vi "CloseNode.vi"(8 "error in":errorcluster, 11 "node ref":T1) -> (0 "error out":errorcluster)   [LabVIEW 2013, in "NISE_CEF_TreeControl.lvlib"]
doc: "This is the node Clean Up Vi it will close all the open references for the node and its childs"
uses:
  NISE_CEF_TreeControl.lvlib
  Node/NodeRef.ctl
  Node/NISE_CEF_Node.lvclass
  Node/NISE_CEF_Node.lvclass/NISE_CEF_Node.ctl
  Node/ReadChildren.vi
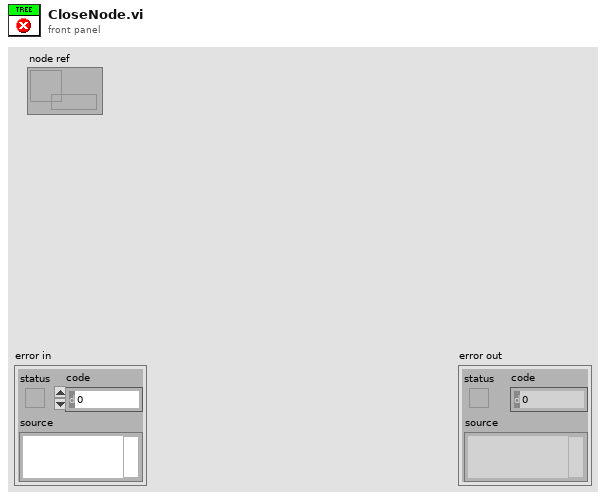
[diagram p1: front panel]
types:
  T1 = typedef "NISE_CEF_Node.lvclass/NodeRef.ctl" = refnum<data-value>
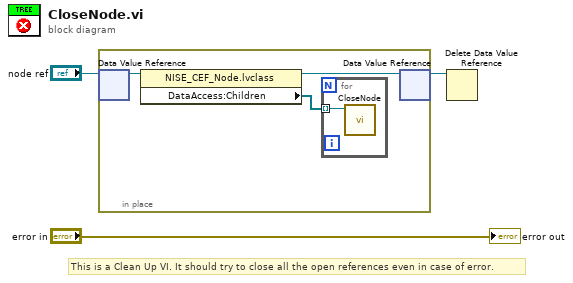
[diagram p0: block diagram]
diagram:
  # "This is a Clean Up VI. It should try to close all the open references even in case of error."
  n1 = in-place {
    n2 = in-place-dvr #1("node ref") -> (w6:refnum<class "NISE_CEF_Node.lvclass">)  [unwired: 1 out]
    n3 = property class="NISE_CEF_Node.lvclass"(reference=w6) -> (reference out=w4:refnum<class "NISE_CEF_Node.lvclass">, "DataAccess:Children"=w5:T1[])  [unwired: 1 in, 1 out]
    n4 = for {
      tunnel: w5 -> [w7] mode=indexing
      n5 = call "CloseNode.vi"("node ref"=w7) -> ()  [unwired: 10 in, 1 out]
    }
    n6 = in-place-dvr #1(w4) -> (w2:T1)  [unwired: 1 out]
  }
  n7 = Delete Data Value Reference(data value reference=w2) -> ()  [unwired: 1 in, 2 out]
  "error out" <- "error in"
